vi "Initialize.vi"(8 "error in (no error)":errorcluster, 9 "Reset (True)":bool=TRUE, 10 "ID Query (True)":bool=TRUE, 11 "VISA resource name":refnum<visa-resource-name>) -> (0 "error out":errorcluster, 3 "VISA resource name out":refnum<visa-resource-name>)   [LabVIEW 2010, in "Agilent 3458.lvlib"]
doc: "Establishes communication with the instrument and optionally performs an instrument identification query and/or an instrument reset. It also places the instrument in a default state needed for other instrument driver operations. Therefore, call this VI before calling other instrument driver VIs for this instrument. Generally, you need to call the Initialize VI only once at the beginning of an application."
uses:
  <instrlib>/Agilent 3458/Agilent 3458.lvlib
panel:
  # "(c) 2007  National Instruments.  ALL RIGHTS RESERVED."
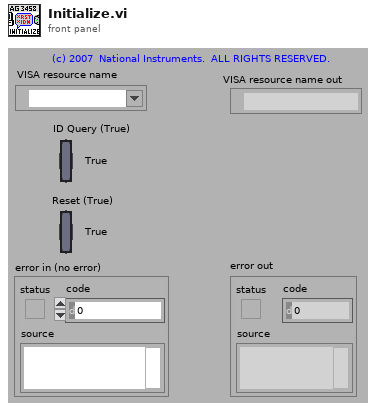
[diagram p1: front panel]
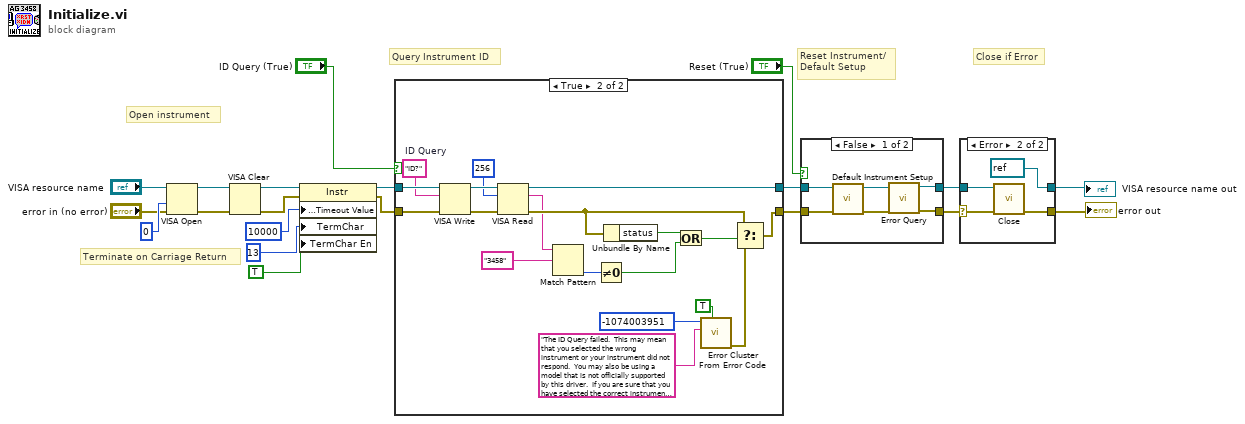
[diagram p0: block diagram]
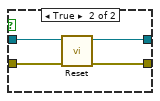
[diagram p3: hidden frame]
diagram:
  # "Terminate on Carriage Return"
  # "Close if Error"
  # "Query Instrument ID"
  # "Reset Instrument/\nDefault Setup"
  # "Open instrument"
  n1 = VISA Open(access mode=u32 0, error in (no error)="error in (no error)", VISA resource name="VISA resource name") -> (VISA resource name=w13:refnum<visa-resource-name>, error out=w12:errorcluster)  [unwired: 2 in]
  n2 = VISA Clear(VISA resource name=w13, error in (no error)=w12) -> (VISA resource name out=w11:refnum<visa-resource-name>, error out=w10:errorcluster)
  n3 = property class="Instr"(reference=w11, error in=w10, "General Settings:Timeout Value"=u32 10000, "TermChar"=u8 13 ("Message Based Settings:Termination Character"), "TermChar En"=TRUE ("Message Based Settings:Termination Character Enable")) -> (reference out=w16:refnum<visa-resource-name>, error out=w15:errorcluster)
  n4 = case shown="True" "ID Query (True)" {
    tunnel: [w21 w41] -> w19
    tunnel: [w22 w38] -> w20
    tunnel: w16 -> [w22 w39]
    tunnel: w15 -> [w21 w40]
    frame False {
    }
    frame True {
      w33 = "ID?"  # ID Query
      n5 = VISA Write(VISA resource name=w39, write buffer=w33, error in (no error)=w40) -> (VISA resource name out=w37:refnum<visa-resource-name>, error out=w36:errorcluster)  [unwired: 1 out]
      n6 = VISA Read(VISA resource name=w37, byte count=u32 256, error in (no error)=w36) -> (VISA resource name out=w38:refnum<visa-resource-name>, read buffer=w24:string, error out=w27:errorcluster)  [unwired: 1 out]
      n7 = Match Pattern(string=w24, regular expression="3458") -> (offset past match=w28:i32)  [unwired: 1 in, 3 out]
      n8 = Not Equal To 0?(x=w28) -> (x != 0?=w23:bool)
      n9 = Unbundle By Name(w27) -> ("status"=w26:bool)
      n10 = Or(x=w26, y=w23) -> (x .or. y?=w25:bool)
      n11 = call <vilib>:"Error Cluster From Error Code.vi"("show call chain? (False)"=TRUE, "error message (\"\")"="The ID Query failed.  This may mean that you selected the wrong instrument or your instrument did not respond.  You may also be using a model that is not officially supported by this driver.  If you are sure that you have selected the correct instrument and it is responding, try disabling the ID Query." ("Source (VI Name)"), "error code (0)"=-1074003951 ("Code")) -> ("error out"=w32:errorcluster)  [unwired: 6 in]
      n12 = Select(t=w27, s=w25, f=w32) -> (s? t:f=w41:errorcluster)
    }
  }
  n13 = case shown="False" "Reset (True)" {
    tunnel: w19 -> [w46 w49]
    tunnel: [w42 w48] -> w8
    tunnel: w20 -> [w47 w50]
    tunnel: [w43 w51] -> w9
    frame False {
      n14 = call <instrlib>:"Default Instrument Setup.vi"("error in (no error)"=w46, "VISA resource name"=w47) -> ("error out"=w44:errorcluster, "VISA resource name out"=w45:refnum<visa-resource-name>)  [unwired: 8 in]
      n15 = call <instrlib>:"Error Query.vi"("error in (no error)"=w44, "VISA resource name"=w45) -> ("error out"=w42:errorcluster, "VISA resource name out"=w43:refnum<visa-resource-name>)  [unwired: 6 in, 2 out]
    }
    frame True {
      n16 = call <instrlib>:"Reset.vi"("error in (no error)"=w49, "VISA resource name"=w50) -> ("error out"=w48:errorcluster, "VISA resource name out"=w51:refnum<visa-resource-name>)  [unwired: 8 in]
    }
  }
  n17 = case shown="Error" w8 {
    selector: w8 -> [w52 w55]
    tunnel: w9 -> [w53 w56]
    tunnel: [w53 refnum<visa-resource-name> refnum ("VISA resource name out")] -> w3
    tunnel: [w52 w57] -> w1
    frame No Error {
    }
    frame Error {
      n18 = call <instrlib>:"Close.vi"("error in (no error)"=w55, "VISA resource name"=w56) -> ("error out"=w57:errorcluster)  [unwired: 9 in]
    }
  }
  "VISA resource name out" <- w3
  "error out" <- w1
